vi "Write Image.vi"(0 "Session In":T1, 1 "Folder":string, 2 "Temp Image Name":string, 3 "Camera Missing?":bool, 5 "Error In":errorcluster, 6 "Student ID":i32, 8 "Student Name":string) -> (14 "Session Out":T1, 16 "Image Out":T2, 19 "Error Out":errorcluster)   [LabVIEW 2017]
uses:
  <vilib>/vision/Image Controls.llb/IMAQ Image.ctl
  <vilib>/userdefined/High Color/IMAQdx.ctl
  <vilib>/vision/driver/NI_Vision_Acquisition_Software.lvlib
panel:
  out "appended path":path
  out "File Path":path
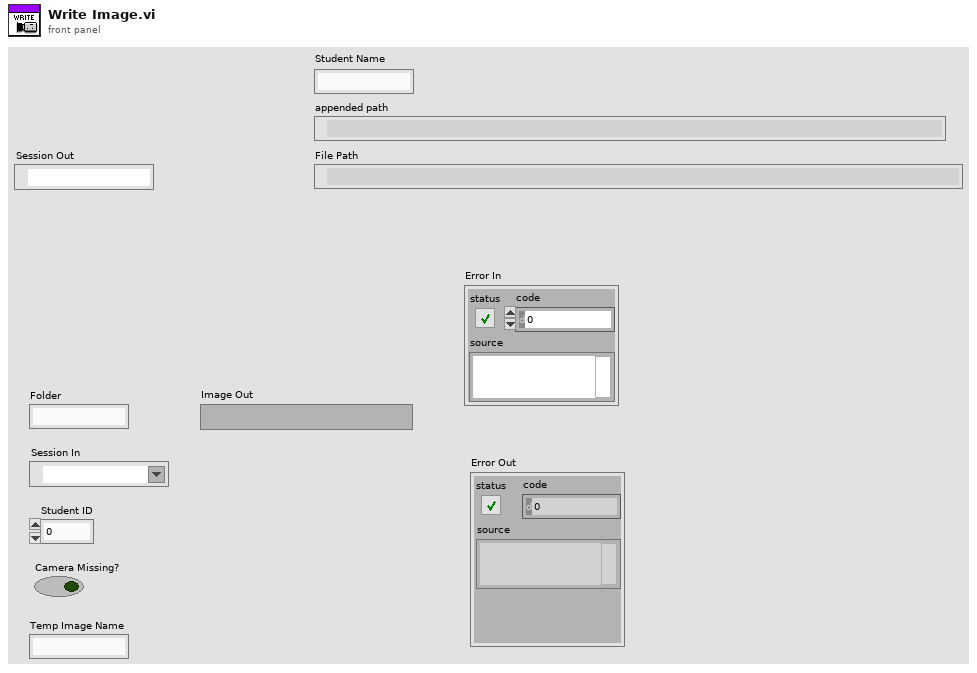
[diagram p1: front panel]
types:
  T1 = typedef "IMAQdx.ctl" = refnum<k21>
  T2 = typedef "IMAQ Image.ctl" = refnum<image>
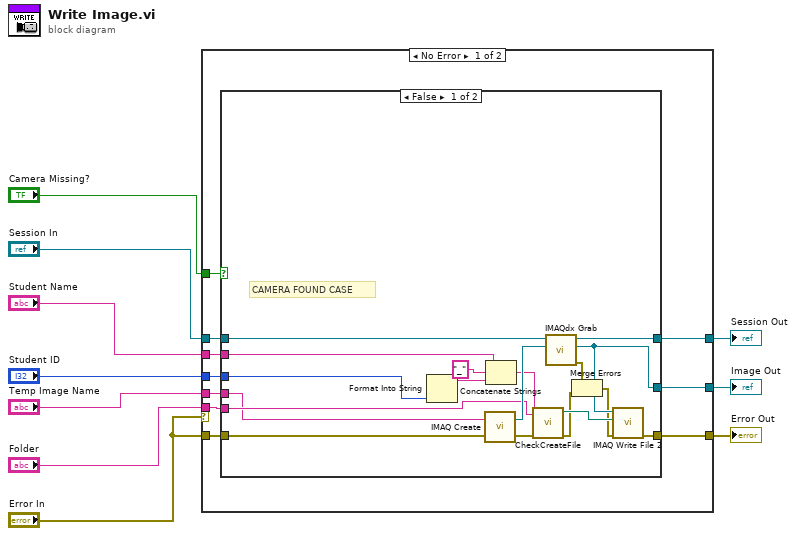
[diagram p0: block diagram]
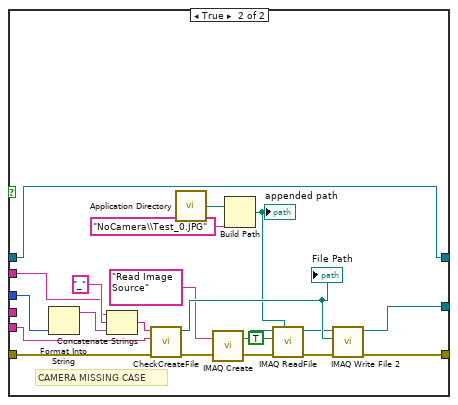
[diagram p2: hidden frame]
diagram:
  n1 = case shown="No Error" "Error In" {
    tunnel: "Student ID" -> [w20 _]
    tunnel: "Camera Missing?" -> [w19 _]
    tunnel: [w18 _] -> w8
    tunnel: "Session In" -> [w17 w60]
    tunnel: [w16 w60] -> w6
    tunnel: [w15 w61] -> w5
    tunnel: "Error In" -> [w14 w61]
    tunnel: "Student Name" -> [w13 _]
    tunnel: "Folder" -> [w12 _]
    tunnel: "Temp Image Name" -> [w11 _]
    frame No Error {
      n2 = case shown="False" w19 {
        tunnel: w17 -> [w38 w54]
        tunnel: [w36 w48] -> w18
        tunnel: w20 -> [w31 w55]
        tunnel: [w30 w54] -> w16
        tunnel: [w29 w45] -> w15
        tunnel: w14 -> [w28 w52]
        tunnel: w13 -> [w26 w39]
        tunnel: w12 -> [w25 w40]
        tunnel: w11 -> [w24 _]
        frame False {
          # "CAMERA FOUND CASE"
          n3 = Format Into String(w31) -> (resulting string=w33:string)  [unwired: 3 in, 1 out]
          n4 = call "IMAQ Create"("Image Name"=w24, "error in (no error)"=w28) -> ("New Image"=w37:T2, "error out"=w27:errorcluster)  [unwired: 2 in, 1 out]
          n5 = Concatenate Strings(w26, "_" ("string"), w33) -> (w32:string)
          n6 = call "CheckCreateFile.vi"("Error In"=w27, "Folder"=w25, "Image Name"=w32) -> ("Error Out"=w22:errorcluster, "File Path"=w35:path)  [unwired: 7 in]
          n7 = call <vilib>:"IMAQdx Grab.vi"("Image In"=w37, "Session In"=w38) -> ("error out"=w23:errorcluster, "Image Out"=w36:T2, "Session Out"=w30:T1)  [unwired: 2 in, 5 out]
          n8 = Merge Errors(w23, w22) -> (w21:errorcluster)
          n9 = call-poly "IMAQ Write File 2"("error in (no error)"=w21, "File Path"=w35, "Image"=w36) -> ("error out"=w29:errorcluster)  [unwired: 7 in, 1 out]
        }
        frame True {
          # "CAMERA MISSING CASE"
          n10 = Format Into String(w55) -> (resulting string=w57:string)  [unwired: 3 in, 1 out]
          n11 = Concatenate Strings(w39, "_" ("string"), w57) -> (w56:string)
          n12 = call "CheckCreateFile.vi"("Error In"=w52, "Folder"=w40, "Image Name"=w56) -> ("Error Out"=w51:errorcluster, "File Path"=w59:path)  [unwired: 7 in]
          "File Path" <- w59
          n13 = call <vilib>:"Application Directory.vi"() -> ("Application Directory"=w44:path)
          n14 = call "IMAQ Create"("Image Name"="Read Image Source", "error in (no error)"=w51) -> ("New Image"=w47:T2, "error out"=w50:errorcluster)  [unwired: 3 in]
          n15 = Build Path(base path=w44, name or relative path="NoCamera\\Test_0.JPG") -> (appended path=w42:path)
          "appended path" <- w42
          n16 = call "IMAQ ReadFile"("File Path"=w42, "error in (no error)"=w50, "Load Color Palette? (No)"=TRUE, "Image"=w47) -> ("error out"=w49:errorcluster, "Image Out"=w46:T2)  [unwired: 3 in, 3 out]
          n17 = call-poly "IMAQ Write File 2"("error in (no error)"=w49, "File Path"=w59, "Image"=w46) -> ("error out"=w45:errorcluster, "Image Out (duplicate)"=w48:T2)  [unwired: 7 in]
        }
      }
    }
    frame Error {
      # "#Replace with Dummy \"Error\" Image"
    }
  }
  "Image Out" <- w8
  "Session Out" <- w6
  "Error Out" <- w5
